vi "Brute Force Measurment SubVI Posibly Modded For Trip Prevention System.vi"(8 "error in (no error)":errorcluster, 9 "BoardHandle in":T1, 11 "Barcodes in":string[](array[string])) -> (0 "Ch 4 High":dbl[](array[numeric]), 1 "Ch 3 High":dbl[](array[numeric]), 2 "Ch 2 High":dbl[](array[numeric]), 3 "Ch 1 High":dbl[](array[numeric]), 4 "error out":errorcluster, 5 "BoardHandle out":T1)   [LabVIEW 2020]
panel:
  # "INPUT"
  # "OUTPUT"
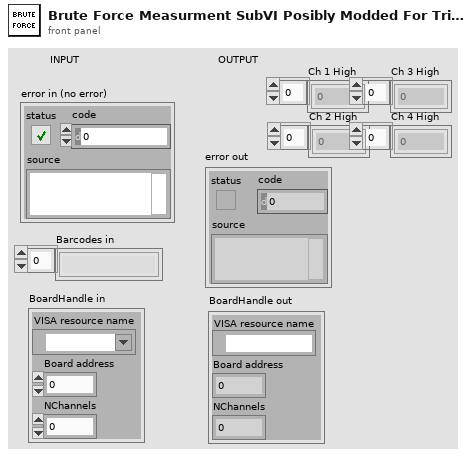
[diagram p1: front panel]
types:
  T1 = cluster{"VISA resource name":refnum<visa-resource-name>, "Board address":u8, "NChannels":u8}
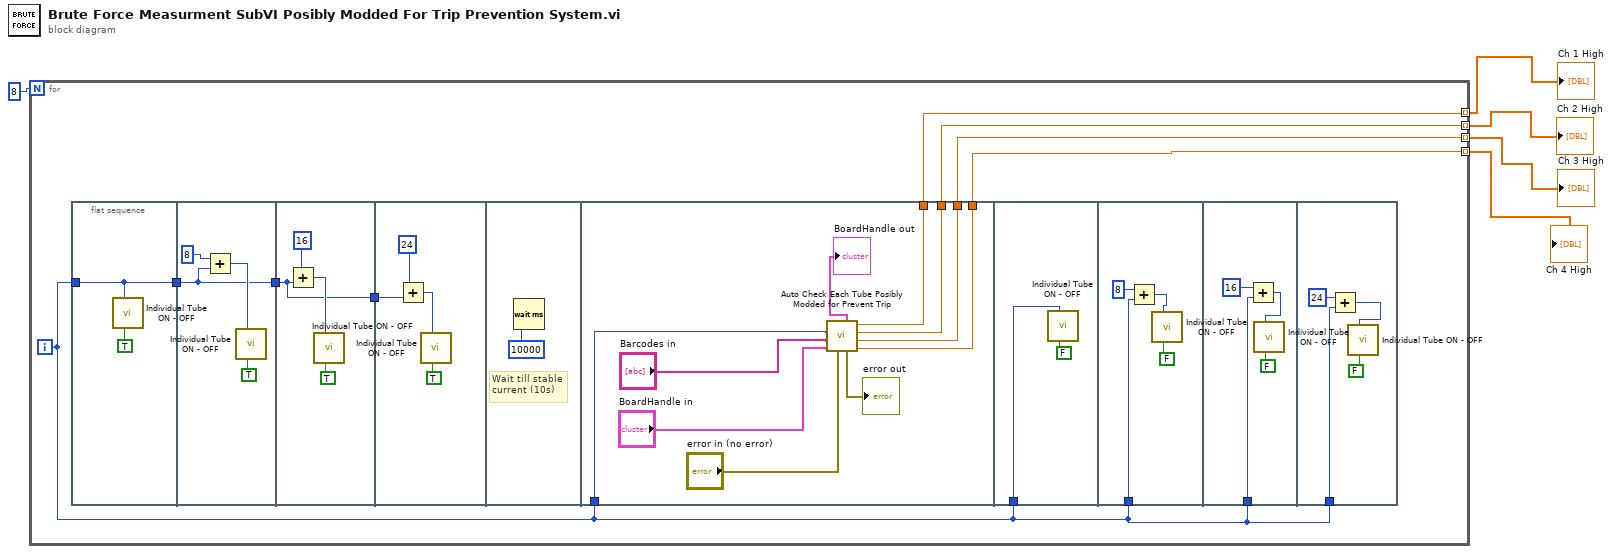
[diagram p0: block diagram]
diagram:
  n1 = for {
    N: 8 -> [_]
    tunnel: [w9] -> w4 mode=indexing
    tunnel: [w8] -> w3 mode=indexing
    tunnel: [w6] -> w2 mode=indexing
    tunnel: [w7] -> w1 mode=indexing
    i -> [w10]
    n2 = flat-sequence {
      tunnel: [w14] -> w13
      tunnel: w10 -> [w14]
      tunnel: w13 -> [w17]
      tunnel: [w17] -> w12
      tunnel: w12 -> [w21]
      tunnel: [w21] -> w11
      tunnel: w11 -> [w25]
      tunnel: w10 -> [w35]
      tunnel: [w32] -> w9
      tunnel: [w31] -> w8
      tunnel: [w30] -> w6
      tunnel: [w29] -> w7
      tunnel: w10 -> [w40]
      tunnel: w10 -> [w43]
      tunnel: w10 -> [w47]
      tunnel: w10 -> [w51]
      frame #0 {
        n3 = call "Individual Tube ON - OFF.vi"("Single Tube ON/OFF"=TRUE, "Tube #"=w14) -> ()  [unwired: 10 in]
      }
      frame #1 {
        n4 = Add(x=8, y=w17) -> (x+y=w19:i32)
        n5 = call "Individual Tube ON - OFF.vi"("Single Tube ON/OFF"=TRUE, "Tube #"=w19) -> ()  [unwired: 10 in]
      }
      frame #2 {
        n6 = Add(x=16, y=w21) -> (x+y=w23:i32)
        n7 = call "Individual Tube ON - OFF.vi"("Single Tube ON/OFF"=TRUE, "Tube #"=w23) -> ()  [unwired: 10 in]
      }
      frame #3 {
        n8 = Add(x=24, y=w25) -> (x+y=w27:i32)
        n9 = call "Individual Tube ON - OFF.vi"("Single Tube ON/OFF"=TRUE, "Tube #"=w27) -> ()  [unwired: 10 in]
      }
      frame #4 {
        # "Wait till stable\ncurrent (10s)"
        n10 = Wait (ms)(milliseconds to wait=u32 10000) -> ()  [unwired: 1 out]
      }
      frame #5 {
        n11 = call "Auto Check Each Tube Posibly Modded for Prevent Trip.vi"("error in (no error)"="error in (no error)", "BoardHandle in"="BoardHandle in", "Barcodes in"="Barcodes in", "Tube #"=w35) -> ("Current 4"=w29:dbl, "Current 3"=w30:dbl, "Current 2"=w31:dbl, "Current 1"=w32:dbl, "error out"=→"error out":errorcluster, "BoardHandle out"=→"BoardHandle out":T1)  [unwired: 2 in]
      }
      frame #6 {
        n12 = call "Individual Tube ON - OFF.vi"("Single Tube ON/OFF"=FALSE, "Tube #"=w40) -> ()  [unwired: 10 in]
      }
      frame #7 {
        n13 = Add(x=8, y=w43) -> (x+y=w44:i32)
        n14 = call "Individual Tube ON - OFF.vi"("Single Tube ON/OFF"=FALSE, "Tube #"=w44) -> ()  [unwired: 10 in]
      }
      frame #8 {
        n15 = Add(x=16, y=w47) -> (x+y=w48:i32)
        n16 = call "Individual Tube ON - OFF.vi"("Single Tube ON/OFF"=FALSE, "Tube #"=w48) -> ()  [unwired: 10 in]
      }
      frame #9 {
        n17 = Add(x=24, y=w51) -> (x+y=w52:i32)
        n18 = call "Individual Tube ON - OFF.vi"("Single Tube ON/OFF"=FALSE, "Tube #"=w52) -> ()  [unwired: 10 in]
      }
    }
  }
  "Ch 1 High" <- w4
  "Ch 2 High" <- w3
  "Ch 3 High" <- w2
  "Ch 4 High" <- w1
